vi "test.ingest_csv_express.vi"() -> ()   [LabVIEW 2020]
uses:
  Nominal Client/Nominal Client.lvclass/Nominal Client.ctl
  nominal types/workspace/workspace.lvclass/workspace.ctl
  ae172e34-dffc-4b12-83ea-48ef3a2c3c44.vi
  f68fde30-30e4-4b08-97bf-6f7da0132bc9.vi
  d999190f-fee9-49b3-afb9-f232f2b660b8.vi
  Nominal Client/private_data.set.vi
  nominal types/workspace/id.get.vi
  nominal types/workspace/rid.get.vi
  <vilib>/AdvancedString/1D String Array to Delimited String.vi
  Nominal Client/workspace.set.vi
  <vilib>/Utility/error.llb/Error Cluster From Error Code.vi
  <vilib>/addons/_JKI.lib/REST Client/classes/REST Client/Create REST Client.vi
  reqwest/NewHttpSession.vi
  Nominal Client/workspace_cache.get_from_rid.vi
  Nominal Client/workspace_cache.get.vi
  Nominal Client/upload_ingest.csv.vi
  Nominal Client/catalog.get_ingest_progress_v2.vi
  reqwest/DestroyHttpSession.vi
  Nominal Client/Nominal Client.lvclass
  nominal types/workspace/workspace.lvclass
  <vilib>/addons/_JKI.lib/REST Client/classes/REST Client/REST Client.lvclass
  reqwest/reQwestClient.lvclass
panel:
  out "Additional Details":T1 {"End Time" format="%<%x %.3X>T"; "Start Time" format="%<%x %.3X>T"}
  out "Status":string
  out "datasetRid":string
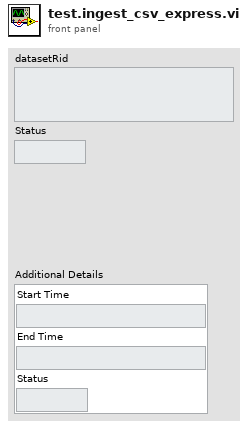
[diagram p1: front panel]
types:
  T1 = cluster{"Start Time":timestamp, "End Time":timestamp, "Status":string}
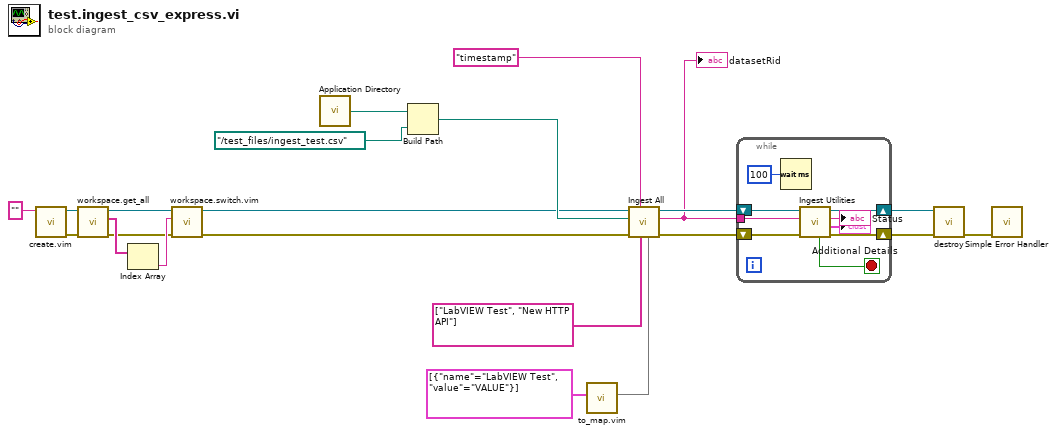
[diagram p0: block diagram]
diagram:
  n1 = call "create.vim"("API Token (string or path)"="") -> ("error out"=w15:errorcluster, "Nominal Client"=w19:refnum<class "Nominal Client.lvclass">)  [unwired: 9 in]
  n2 = call "workspace.get_all.vi"("error in"=w15, "Nominal Client in"=w19) -> ("error out"=w14:errorcluster, "Workspace RIDs"=w17:string[], "Nominal Client out"=w18:refnum<class "Nominal Client.lvclass">)  [unwired: 5 in, 2 out]
  n3 = Index Array(array=w17) -> (element=w16:string)  [unwired: 1 in]
  n4 = call "workspace.switch.vim"("error in"=w14, "Workspace RID (string or path)"=w16, "Nominal Client in"=w18) -> ("error out"=w1:errorcluster, "Nominal Client out"=w2:refnum<class "Nominal Client.lvclass">)  [unwired: 7 in]
  n5 = call <vilib>:"Application Directory.vi"() -> ("Application Directory"=w21:path)
  n6 = Build Path(base path=w21, name or relative path=path "../test_files/ingest_test.csv") -> (appended path=w5:path)
  n7 = call "to_map.vim"("Map"=cluster{"name":string, "value":string}[] [{"name"="LabVIEW Test", "value"="VALUE"}] ("properties")) -> ("Map out"=w3:map{string, string})  [unwired: 10 in]
  n8 = call-poly "Ingest All.vi"("Properties"=w3, "Labels"=string[] ["LabVIEW Test", "New HTTP API"] ("labels"), "Timestamp SeriesName"="timestamp" ("seriesName"), "error in"=w1, "File Path"=w5, "Nominal Client in"=w2) -> ("error out"=w10:errorcluster, "datasetRID"=w9:string, "Nominal Client out"=w11:refnum<class "Nominal Client.lvclass">)  [unwired: 3 in]
  "datasetRid" <- w9
  n9 = while {
    tunnel: w9 -> [w29]
    shift-right: [w28] -> w7
    shift-left: w11 -> [w31]
    shift-right: [w27] -> w8
    shift-left: w10 -> [w30]
    stop <- w23 stop-if-true
    n10 = Wait (ms)(milliseconds to wait=u32 100) -> ()  [unwired: 1 out]
    n11 = call-poly "Ingest Utilities.vi"("error in"=w30, "datasetRid[]"=w29, "Nominal Client in"=w31) -> ("error out"=w27:errorcluster, "Additional Details"=→"Additional Details":T1, "Status"=→"Status":string, "Nominal Client out"=w28:refnum<class "Nominal Client.lvclass">, "Complete"=w23:bool)  [unwired: 4 in]
  }
  n12 = call "destroy.vi"("error in"=w8, "Nominal Client"=w7) -> ("error out"=w12:errorcluster)  [unwired: 9 in]
  n13 = call <vilib>:"Simple Error Handler.vi"("error in (no error)"=w12) -> ()  [unwired: 4 in, 5 out]
